vi "HandleSize Test.vi"() -> ()   [LabVIEW 2020]
panel:
  out "size":u64
  out "error out":errorcluster
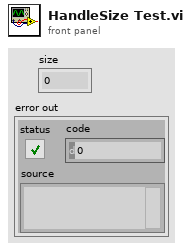
[diagram p1: front panel]
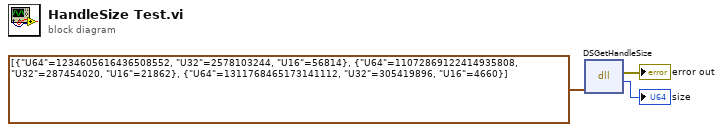
[diagram p0: block diagram]
diagram:
  n1 = dll-call lib="LabVIEW" fn="DSGetHandleSize"("handle"=cluster{"U64":u64, "U32":u32, "U16":u16}[] [{"U64"=1234605616436508552, "U32"=2578103244, "U16"=56814}, {"U64"=11072869122414935808, "U32"=287454020, "U16"=21862}, {"U64"=1311768465173141112, "U32"=305419896, "U16"=4660}]) -> (error out=→"error out":errorcluster, "return type"=→"size":u64)  [unwired: 4 in, 1 out]
